vi "daytime.vi"(2 "Daytime end":timestamp=timestamp(-14400 s since 1904-01-01) format="%<%I:%M %p>T", 3 "Daytime start":timestamp=timestamp(-46800 s since 1904-01-01) format="%<%I:%M %p>T") -> (0 "Mode of day":enum16{"day", "night"}(ring), 1 "Time Stamp":timestamp=timestamp(18000 s since 1904-01-01) format="%<%I:%M:%S %p>T")   [LabVIEW 2021]
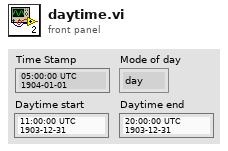
[diagram p1: front panel]
types:
  T1 = typedef "LVDateTimeRec.ctl" = cluster{"fractional second":dbl, "second":i32, "minute":i32, "hour":i32, "day of month":i32, "month":i32, "year":i32, "day of week":i32, "day of year":i32, "DST":i32}
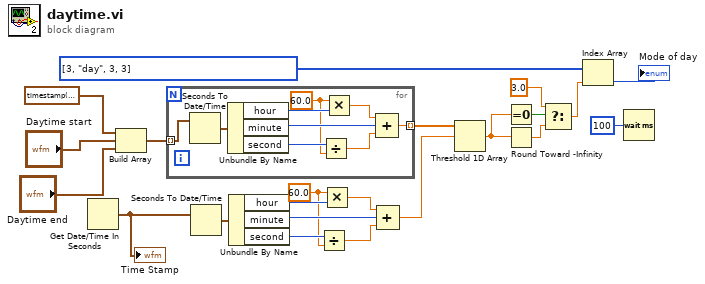
[diagram p0: block diagram]
diagram:
  w15 = 60.0 ("x")
  w22 = enum16{"day", "night"}[] [3, enum."day", 3, 3] items=["day", "night"]
  n1 = Get Date/Time In Seconds() -> (seconds since 1Jan1904=w6:timestamp)
  "Time Stamp" <- w6
  n2 = Build Array(timestamp(-68400 s since 1904-01-01) ("new element/subarray"), "Daytime start", "Daytime end") -> (w2:timestamp[])
  n3 = for {
    tunnel: [w24] -> w21 mode=indexing
    tunnel: w2 -> [w23] mode=indexing
    w26 = 60.0 ("x")
    n4 = Seconds To Date/Time(time stamp (now)=w23) -> (date time rec=w31:T1)  [unwired: 1 in]
    n5 = Unbundle By Name(w31) -> ("hour"=w30:i32, "minute"=w28:i32, "second"=w27:i32)
    n6 = Divide(x=w27, y=w26) -> (x/y=w25:dbl)
    n7 = Multiply(x=w26, y=w30) -> (x*y=w29:dbl)
    n8 = Compound Arithmetic op=ADD(w29, w28, w25) -> (w24:dbl)
  }
  n9 = Seconds To Date/Time(time stamp (now)=w6) -> (date time rec=w20:T1)  [unwired: 1 in]
  n10 = Unbundle By Name(w20) -> ("hour"=w19:i32, "minute"=w17:i32, "second"=w16:i32)
  n11 = Divide(x=w16, y=w15) -> (x/y=w14:dbl)
  n12 = Multiply(x=w15, y=w19) -> (x*y=w18:dbl)
  n13 = Compound Arithmetic op=ADD(w18, w17, w14) -> (w13:dbl)
  n14 = Threshold 1D Array(2:w13, 3:w21) -> (0:w8:dbl)  [unwired: 1 in]
  n15 = Equal To 0?(x=w8) -> (x = 0?=w7:bool)
  n16 = Round Toward -Infinity(1:w8) -> (0:w10:dbl)
  n17 = Select(t=3.0, s=w7, f=w10) -> (s? t:f=w9:dbl)
  n18 = Index Array(array=w22, index=w9) -> (element=→"Mode of day":enum16{"day", "night"})
  n19 = Wait (ms)(milliseconds to wait=u32 100) -> ()  [unwired: 1 out]
